vi "Global Lookup.vi"(8 "Read(f) Write(T)":bool, 9 "Value":u64, 11 "Key":T1) -> (1 "Value Out":u64, 3 "Key Found Out":bool)   [LabVIEW 2023]
uses:
  Cluster Array Key.ctl
  ENUM_Type.ctl
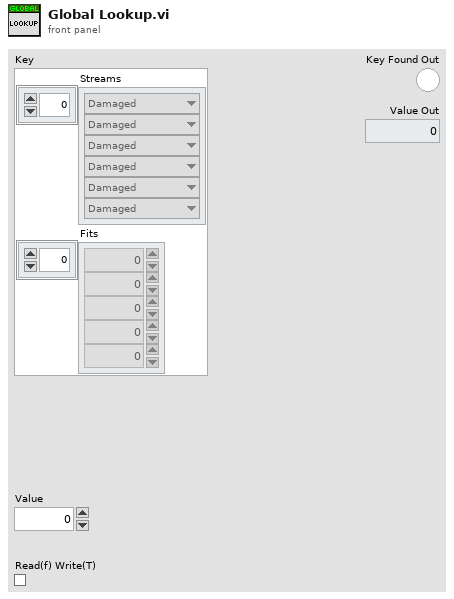
[diagram p1: front panel]
types:
  T1 = typedef "Cluster Array Key.ctl" = cluster{"Streams":T2[], "Fits":i32[]}
  T2 = typedef "ENUM_Type.ctl" = enum16{"Damaged", "Operational", "Unknown"}
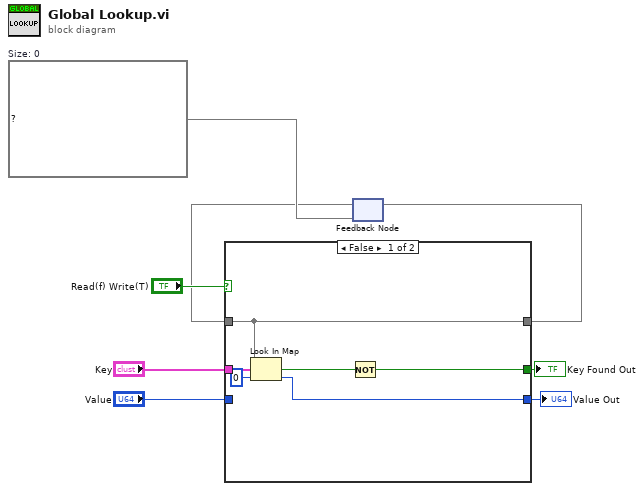
[diagram p0: block diagram]
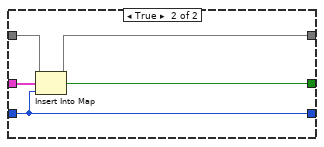
[diagram p2: hidden frame]
diagram:
  w7 = map{T1, u64} {}  # Size: 0
  n1 = feedback #1(w7) -> (w2:map{T1, u64})
  n2 = case shown="False" "Read(f) Write(T)" {
    tunnel: w2 -> [w13 w19]
    tunnel: "Key" -> [w14 w18]
    tunnel: "Value" -> [_ w17]
    tunnel: [w10 w17] -> w4
    tunnel: [w13 w16] -> w3
    tunnel: [w11 w15] -> w1
    frame False {
      n3 = Look In Map(map=w13, key=w14, default value=u64 0) -> (key not found?=w12:bool, value=w10:u64)
      n4 = Not(x=w12) -> (.not. x?=w11:bool)
    }
    frame True {
      n5 = Insert Into Map(map in=w19, key=w18, value=w17) -> (map out=w16:map{T1, u64}, key already included?=w15:bool)  [unwired: 1 out]
    }
  }
  "Value Out" <- w4
  "Key Found Out" <- w1
  n6 = feedback-in #1(w3) -> ()
